vi "Is Support Pre Trigger Percent.vi"(8 "error in (no error)":errorcluster) -> (0 "error out":errorcluster, 3 "function return":bool)   [LabVIEW 2021, in "vmmsolib.lvlib"]
doc: "DLL_API bool WINAPI IsSupportPreTriggerPercent();"
uses:
  vmmsolib.lvlib
  vmmso.dll
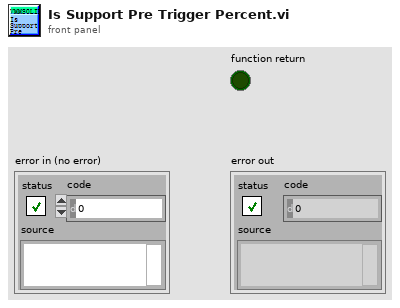
[diagram p1: front panel]
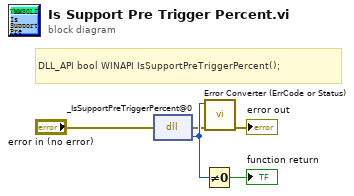
[diagram p0: block diagram]
diagram:
  # "DLL_API bool WINAPI IsSupportPreTriggerPercent();"
  n1 = dll-call lib="D:/VmMsoSDK/demo-Labview/2021/vmmsolib/vmmso.*" fn="_IsSupportPreTriggerPercent@0"(error in="error in (no error)") -> (error out=w2:errorcluster, w4:u8)  [unwired: 2 in, 1 out]
  n2 = Not Equal To 0?(x=w4) -> (x != 0?=→"function return":bool)
  n3 = call "Error Converter (ErrCode or Status).vi"("error in (no error)"=w2, "error code"=w4) -> ("error out"=→"error out":errorcluster)  [unwired: 9 in]
